vi "Climb_Execute.vi"() -> ()   [LabVIEW 2018]
uses:
  <vilib>/Rock Robotics/WPI/ThirdParty/Phoenix-LabVIEW/Motor Controller/Controls/CTRE_Phoenix_MotorControl_ControlMode.ctl
  <vilib>/Rock Robotics/WPI/Solenoid/WPI_SolenoidValue.ctl
  Global_Variables/Climb_Globals.vi
  <vilib>/Rock Robotics/WPI/Solenoid/WPI_SolenoidGetEnum.vi
  Global_Variables/Sensor_Values.vi
  <vilib>/Rock Robotics/WPI/Solenoid/WPI_SolenoidSetEnum.vi
panel:
  in  "Speed_Down":dbl=-0.3 format="%#_13g"
  in  "Drop_Pos":dbl=2500.0
  in  "Climb_Gain":dbl=0.00012
  in  "Gain":dbl=1e-06
  in  "Backward_Speed":dbl=-1.0
  in  "Forward_Speed":dbl=1.0
  in  "Down_Speed":dbl=-0.3
  in  "Up_Speed":dbl=0.2
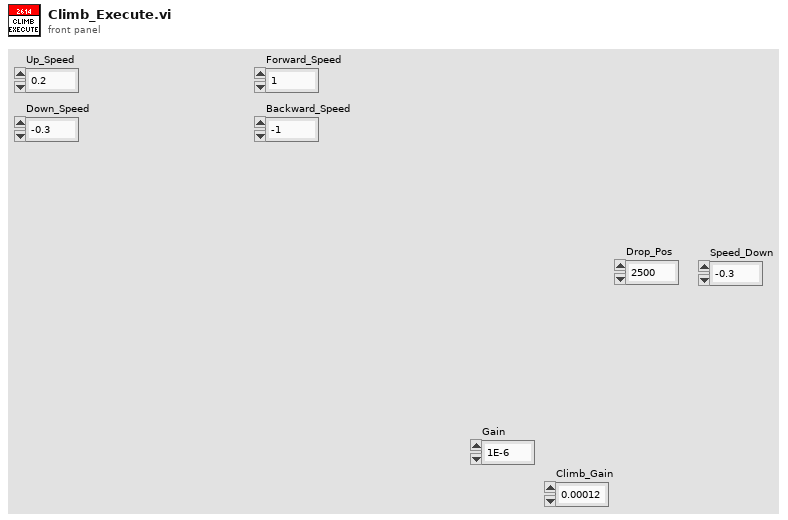
[diagram p1: front panel]
types:
  T1 = typedef "WPI_SolenoidDevRef.ctl" = cluster{"DevStatus":errorcluster, "Pneumatics Control Module":u8, "Forward Solenoid Channel":T2, "Reverse Solenoid Channel":T2}
  T2 = typedef "WPI_SolenoidChannel.ctl" = enum8{"Solenoid 0", "Solenoid 1", "Solenoid 2", "Solenoid 3", "Solenoid 4", "Solenoid 5", "Solenoid 6", "Solenoid 7", "Invalid"}
  T3 = typedef "WPI_SolenoidValue.ctl" = enum16{"Off", "On", "Forward", "Reverse"}
  T4 = typedef "WPI_MotorControlDeviceRef.ctl" = cluster{"DeviceStatus":errorcluster, "Type":T5, "PWM":cluster{"PWM Channel":T6, "DeadBand":T7}, "CAN":cluster{"Device Number":u8, "SetOutput VI Ref":variant, "GetOutput VI Ref":variant, "Enable VI Ref":variant, "Disable VI Ref":variant, "Data":variant}, "Invert":bool, "DIO PWM":cluster{"PWM \"Enable\" Channel":T6, "DIOChannel":T8, "PWM Rate":dbl}}
  T5 = typedef "WPI_MotorControlType.ctl" = enum16{"PWM", "CAN", "DIO PWM"}
  T6 = typedef "FPGA_DIOPWMChannel.ctl" = enum8{"PWM 0", "PWM 1", "PWM 2", "PWM 3", "PWM 4", "PWM 5", "PWM 6", "PWM 7", "PWM 8", "PWM 9", "PWM MXP 0", "PWM MXP 1", "PWM MXP 2", "PWM MXP 3", "PWM MXP 4", "PWM MXP 5", "PWM MXP 6", "PWM MXP 7", "PWM MXP 8", "PWM MXP 9", "Invalid"}
  T7 = typedef "WPI_PWMDeadband.ctl" = cluster{"Name":string, "maxPositivePwm":i32, "minPositivePwm":i32, "centerPwm":i32, "maxNegativePwm":i32, "minNegativePwm":i32, "angularRange":u16}
  T8 = typedef "FPGA_DIOChannel.ctl" = enum8{"DIO 0", "DIO 1", "DIO 2", "DIO 3", "DIO 4", "DIO 5", "DIO 6", "DIO 7", "DIO 8", "DIO 9", "DIO MXP 0", "DIO MXP 1", "DIO MXP 2", "DIO MXP 3", "DIO MXP 4", "DIO MXP 5", "DIO MXP 6", "DIO MXP 7", "DIO MXP 8", "DIO MXP 9", "DIO MXP 10", "DIO MXP 11", "DIO MXP 12", "DIO MXP 13", "DIO MXP 14", "DIO MXP 15", "SPI Port CS1", "SPI Port CS2", "SPI Port CS3", "SPI Port MISO", "SPI Port MOSI", "Invalid"}
  T9 = typedef "WPI_ServoDeviceRef.ctl" = cluster{"DeviceStatus":errorcluster, "PWM Channel":T6, "DeadBand":T7}
  T10 = typedef "Climb_Notifier.ctl" = cluster{"Climb_Control_Type":T11, "Brake":bool, "Manual_Climb_Up":bool, "Manual_Drive_Forward":bool, "Manual_Drive_Backward":bool, "Manual_Climb_Down":bool, "Climb_Advance":bool, "Climb_Reverse":bool, "Parameter_One":dbl, "Parameter_Two":dbl, "Parameter_Three":dbl, "Step":i32, "Climb_Notifier":refnum<notifier>, "Climb_Distance":dbl, "Level_Two":bool, "Brake_State":bool, "Toggle_Servo":bool, "Drop_Back":bool}
  T11 = typedef "Climb_Control_Type.ctl" = enum16{"No_Op", "Brake", "Manual_Climb_Up", "Manual_Climb_Down", "Manual_Drive_Forward", "Manual_Drive_Backward", "Back_Wheels_Forward", "Lift_Retract", "Lift_Extend", "Extend_to_Second_Level", "Drop_Down", "Spin"}
  T12 = typedef "CTRE_Phoenix_MotorControl_ControlMode.ctl" = u16
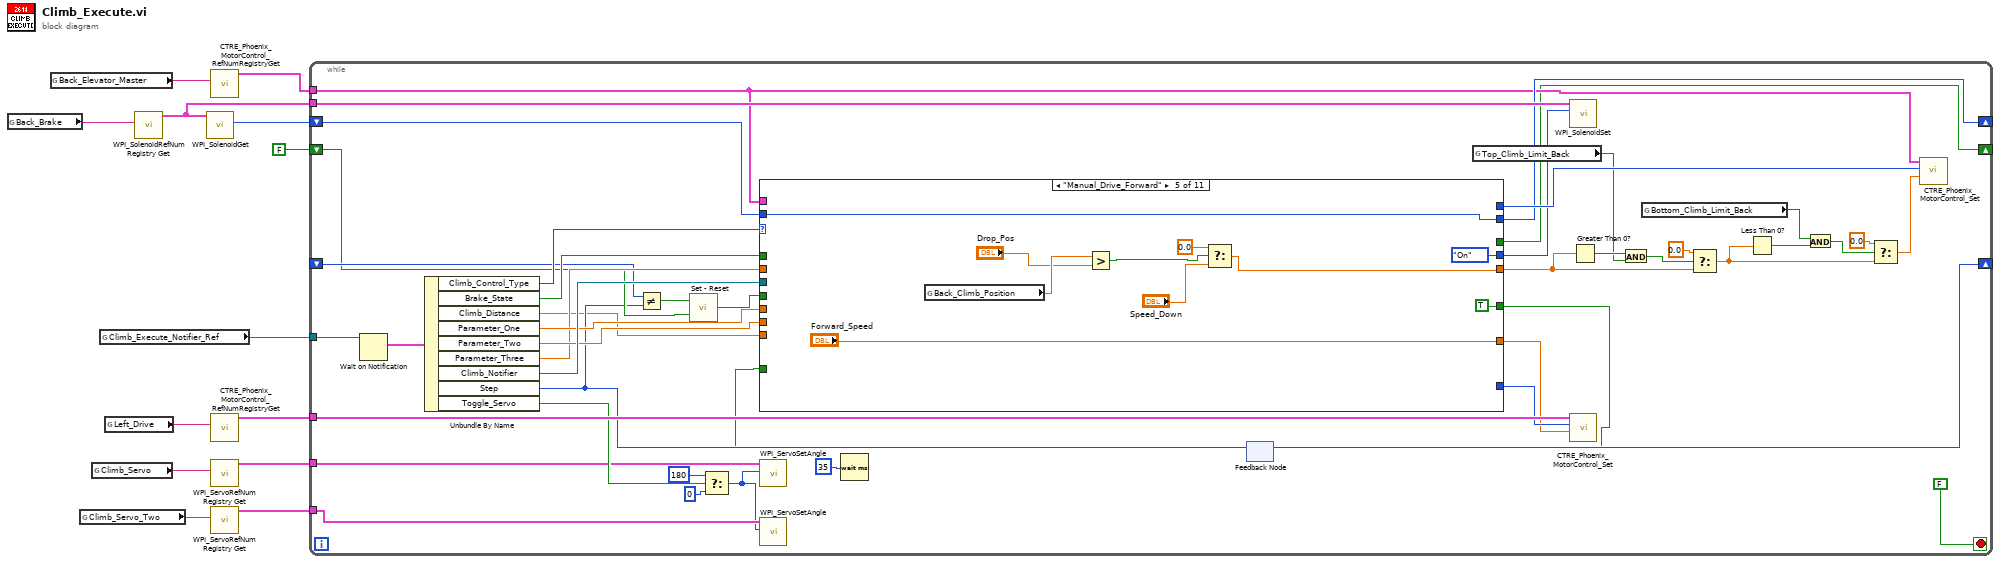
[diagram p0: block diagram]
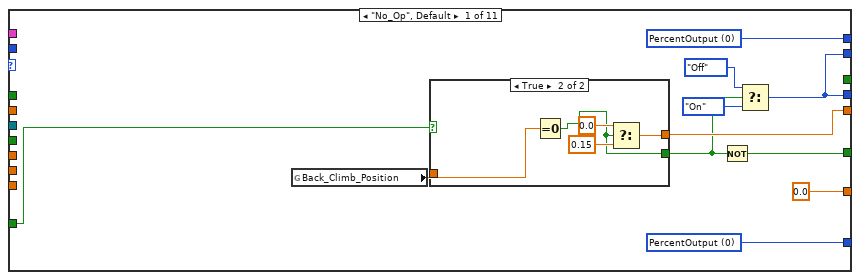
[diagram p2: hidden frame]
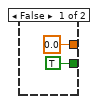
[diagram p3: hidden frame]
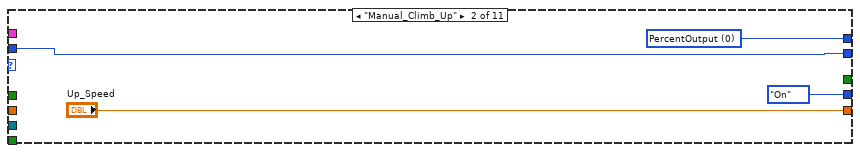
[diagram p4: hidden frame]
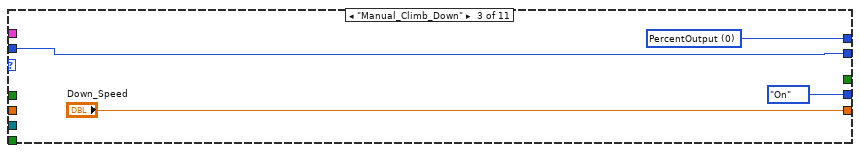
[diagram p5: hidden frame]
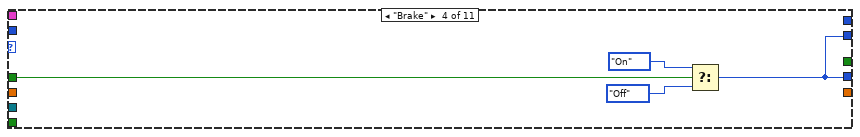
[diagram p6: hidden frame]
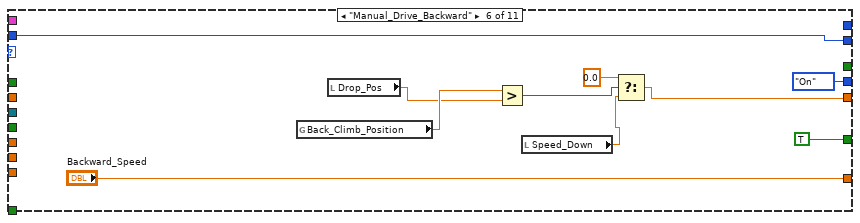
[diagram p7: hidden frame]
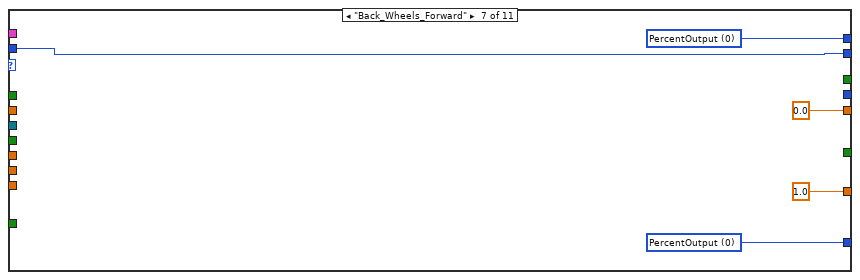
[diagram p8: hidden frame]
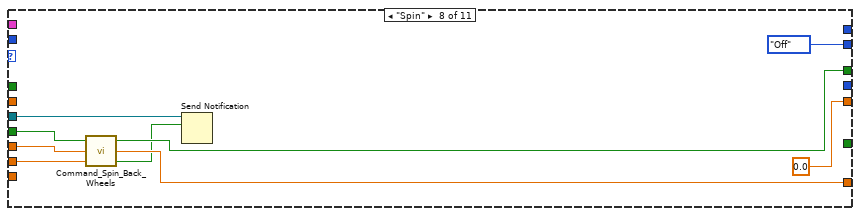
[diagram p9: hidden frame]
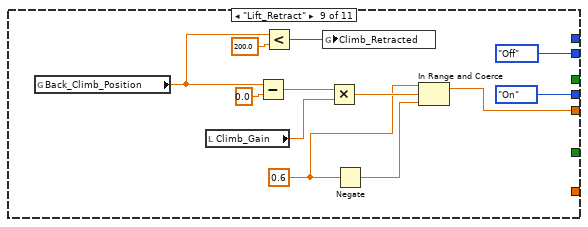
[diagram p10: hidden frame]
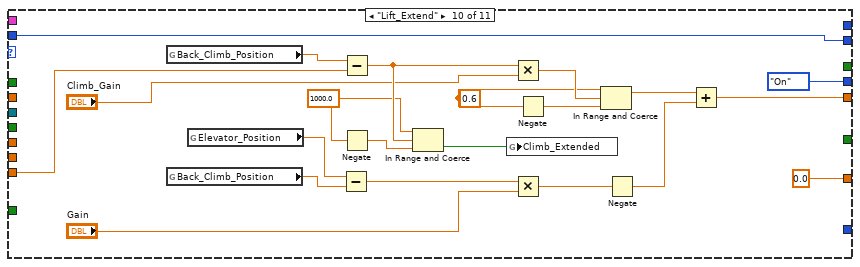
[diagram p11: hidden frame]
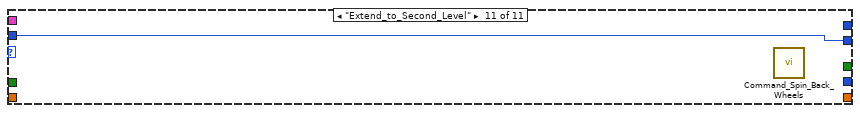
[diagram p12: hidden frame]
diagram:
  n1 = global read "Climb_Globals.vi" "Back_Brake"() -> (w8:string)
  n2 = global read "Climb_Globals.vi" "Back_Elevator_Master"() -> (w11:string)
  n3 = global read "Climb_Globals.vi" "Climb_Servo_Two"() -> (w2:string)
  n4 = global read "Climb_Globals.vi" "Climb_Servo"() -> (w3:string)
  n5 = global read "Climb_Globals.vi" "Climb_Execute_Notifier_Ref"() -> (w12:refnum<notifier>)
  n6 = global read "Climb_Globals.vi" "Left_Drive"() -> (w10:string)
  n7 = call <vilib>:"WPI_SolenoidRefNum Registry Get.vi"("refnum name"=w8) -> ("SolenoidDevRef"=w5:T1)  [unwired: 9 in, 1 out]
  n8 = call-poly <vilib>:"WPI_SolenoidGet.vi"("SolenoidDevRef"=w5) -> ("Value"=w6:T3)  [unwired: 8 in, 2 out]
  n9 = call <vilib>:"CTRE_Phoenix_MotorControl_RefNumRegistryGet.vi"("refnum name"=w11) -> ("PhoenixMotorControlDevRef"=w13:T4)  [unwired: 9 in, 1 out]
  n10 = call <vilib>:"CTRE_Phoenix_MotorControl_RefNumRegistryGet.vi"("refnum name"=w10) -> ("PhoenixMotorControlDevRef"=w9:T4)  [unwired: 9 in, 1 out]
  n11 = call <vilib>:"WPI_ServoRefNum Registry Get.vi"("refnum name"=w3) -> ("ServoDeviceRef"=w4:T9)  [unwired: 9 in, 1 out]
  n12 = call <vilib>:"WPI_ServoRefNum Registry Get.vi"("refnum name"=w2) -> ("ServoDeviceRef"=w1:T9)  [unwired: 9 in, 1 out]
  n13 = while {
    tunnel: w12 -> [w56]
    tunnel: w13 -> [w35]
    tunnel: w9 -> [w53]
    tunnel: w5 -> [w51]
    shift-right: [w49] -> _
    shift-left: w6 -> [w48]
    shift-right: [w25] -> _
    shift-left: _ -> [w28]
    shift-right: [w23] -> _
    shift-left: FALSE -> [w26]
    tunnel: w4 -> [w19]
    tunnel: w1 -> [w17]
    stop <- FALSE stop-if-true
    n14 = Wait on Notification(notifier=w56) -> (notification=w55:T10)  [unwired: 3 in, 3 out]
    n15 = Unbundle By Name(w55) -> ("Climb_Control_Type"=w33:T11, "Brake_State"=w47:bool, "Climb_Distance"=w22:dbl, "Parameter_One"=w31:dbl, "Parameter_Two"=w30:dbl, "Parameter_Three"=w29:dbl, "Climb_Notifier"=w32:refnum<notifier>, "Step"=w25:i32, "Toggle_Servo"=w21:bool)
    n16 = Not Equal?(x=w28, y=w25) -> (x != y?=w27:bool)
    n17 = call "Set - Reset.vi"("Reset"=w26, "Set"=w27) -> ("Output"=w24:bool)
    n18 = Select(t=180, s=w21, f=0 ("Angle")) -> (s? t:f=w16:i32)
    n19 = call <vilib>:"WPI_ServoSetAngle.vi"("Angle"=w16, "ServoDeviceRef"=w19) -> ()  [unwired: 8 in, 2 out]
    n20 = call <vilib>:"WPI_ServoSetAngle.vi"("Angle"=w16, "ServoDeviceRef"=w17) -> ()  [unwired: 8 in, 2 out]
    n21 = Wait (ms)(milliseconds to wait=u32 35) -> ()  [unwired: 1 out]
    n22 = feedback #1() -> (w14:bool)  [unwired: 1 in]
    n23 = case shown="\"Manual_Drive_Forward\"" w33 {
      tunnel: [w69 w78 w82 _ _ _ w112 _ _ _ _] -> w54
      tunnel: [w68 _ _ _ _ _ w111 _ _ _ _] -> w52
      tunnel: [0.0 ("Output") _ _ _ "Forward_Speed" "Backward_Speed" 1.0 ("Speed") w118 _ 0.0 ("Speed") _] -> w38
      tunnel: [w63 WPI_SolenoidValue."On" ("Value") WPI_SolenoidValue."On" ("Value") w86 WPI_SolenoidValue."On" ("Value") WPI_SolenoidValue."On" ("Value") _ _ WPI_SolenoidValue."On" ("Value") WPI_SolenoidValue."On" ("Value") _] -> w50
      tunnel: w47 -> [_ _ _ w85 _ _ _ _ _ _ _]
      tunnel: [w63 w80 w84 w86 w97 w107 w113 WPI_SolenoidValue."Off" ("Value") WPI_SolenoidValue."Off" ("Value") w136 w156] -> w49
      tunnel: w48 -> [_ w80 w84 _ w97 w107 w113 _ _ w136 w156]
      tunnel: w35 -> [_ _ _ _ _ _ _ _ _ _ _]
      tunnel: [w65 "Up_Speed" "Down_Speed" _ w94 w105 0.0 ("upper limit") 0.0 ("upper limit") w125 w142 _] -> w34
      tunnel: w32 -> [_ _ _ _ _ _ _ w114 _ _ _]
      tunnel: w31 -> [_ _ _ _ _ _ _ w121 _ _ _]
      tunnel: w30 -> [_ _ _ _ _ _ _ w120 _ _ _]
      tunnel: w29 -> [_ _ _ _ _ _ _ _ _ _ _]
      tunnel: w24 -> [_ _ _ _ _ _ _ w119 _ _ _]
      tunnel: [_ _ _ _ _ _ _ w116 _ _ _] -> w23
      tunnel: w22 -> [_ _ _ _ _ _ _ _ _ w135 _]
      tunnel: [w59 _ _ _ TRUE TRUE _ _ _ _ _] -> w15
      tunnel: w14 -> [w64 _ _ _ _ _ _ _ _ _ _]
      frame "No_Op", Default {
        w68 = T12 0 items=["PercentOutput"=0, "Position"=1, "Velocity"=2, "Current"=3, "Follower"=5, "MotionProfile"=6, "MotionMagic"=7, "MotionProfileArc"=10, "Disabled"=15] ("Control Mode")
        w69 = T12 0 items=["PercentOutput"=0, "Position"=1, "Velocity"=2, "Current"=3, "Follower"=5, "MotionProfile"=6, "MotionMagic"=7, "MotionProfileArc"=10, "Disabled"=15] ("Control Mode")
        n24 = global read "Sensor_Values.vi" "Back_Climb_Position"() -> (w66:dbl)
        n25 = case shown="True" w64 {
          tunnel: w66 -> [_ w73]
          tunnel: [0.0 ("f") w74] -> w65
          tunnel: [TRUE w72] -> w62
          frame False {
          }
          frame True {
            n26 = Equal To 0?(x=w73) -> (x = 0?=w72:bool)
            n27 = Select(t=0.0, s=w72, f=0.15) -> (s? t:f=w74:dbl)
          }
        }
        n28 = Not(x=w62) -> (.not. x?=w59:bool)
        n29 = Select(t=WPI_SolenoidValue."Off" ("Value"), s=w62, f=WPI_SolenoidValue."On") -> (s? t:f=w63:T3)
      }
      frame "Manual_Climb_Up" {
        w78 = T12 0 items=["PercentOutput"=0, "Position"=1, "Velocity"=2, "Current"=3, "Follower"=5, "MotionProfile"=6, "MotionMagic"=7, "MotionProfileArc"=10, "Disabled"=15] ("Control Mode")
      }
      frame "Manual_Climb_Down" {
        w82 = T12 0 items=["PercentOutput"=0, "Position"=1, "Velocity"=2, "Current"=3, "Follower"=5, "MotionProfile"=6, "MotionMagic"=7, "MotionProfileArc"=10, "Disabled"=15] ("Control Mode")
      }
      frame "Brake" {
        n30 = Select(t=WPI_SolenoidValue."On" ("Value"), s=w85, f=WPI_SolenoidValue."Off" ("Value")) -> (s? t:f=w86:T3)
      }
      frame "Manual_Drive_Forward" {
        n31 = global read "Sensor_Values.vi" "Back_Climb_Position"() -> (w91:dbl)
        n32 = Greater?(x=w91, y="Drop_Pos") -> (0:w89:bool)
        n33 = Select(t=0.0, s=w89, f="Speed_Down") -> (s? t:f=w94:dbl)
      }
      frame "Manual_Drive_Backward" {
        n34 = global read "Sensor_Values.vi" "Back_Climb_Position"() -> (w101:dbl)
        n35 = local read "Drop_Pos"() -> (w99:dbl)
        n36 = Greater?(x=w101, y=w99) -> (0:w100:bool)
        n37 = local read "Speed_Down"() -> (w102:dbl)
        n38 = Select(t=0.0, s=w100, f=w102) -> (s? t:f=w105:dbl)
      }
      frame "Back_Wheels_Forward" {
        w111 = T12 0 items=["PercentOutput"=0, "Position"=1, "Velocity"=2, "Current"=3, "Follower"=5, "MotionProfile"=6, "MotionMagic"=7, "MotionProfileArc"=10, "Disabled"=15] ("Control Mode")
        w112 = T12 0 items=["PercentOutput"=0, "Position"=1, "Velocity"=2, "Current"=3, "Follower"=5, "MotionProfile"=6, "MotionMagic"=7, "MotionProfileArc"=10, "Disabled"=15] ("Control Mode")
      }
      frame "Spin" {
        n39 = call "Command_Spin_Back_Wheels.vi"("Timeout"=w120, "Speed"=w121, "Startup"=w119) -> ("Completed"=w115:bool, "Speed_Out"=w118:dbl, "Reinit"=w116:bool)
        n40 = Send Notification(notification=w115, notifier=w114) -> ()  [unwired: 1 in, 2 out]
      }
      frame "Lift_Retract" {
        w129 = 0.6 ("upper limit")
        n41 = global read "Sensor_Values.vi" "Back_Climb_Position"() -> (w127:dbl)
        n42 = local read "Climb_Gain"() -> (w133:dbl)
        n43 = Subtract(x=w127, y=0.0) -> (x-y=w134:dbl)
        n44 = Less?(x=w127, y=200.0) -> (x < y?=w126:bool)
        n45 = global write "Climb_Globals.vi" "Climb_Retracted"(w126) -> ()
        n46 = Multiply(x=w134, y=w133) -> (x*y=w132:dbl)
        n47 = Negate(x=w129) -> (-x=w131:dbl)
        n48 = In Range and Coerce(upper limit=w129, x=w132, lower limit=w131) -> (coerced(x)=w125:dbl)  [unwired: 1 out]
      }
      frame "Lift_Extend" {
        w140 = 1000.0 ("upper limit")
        w139 = 0.6 ("upper limit")
        n49 = global read "Sensor_Values.vi" "Back_Climb_Position"() -> (w153:dbl)
        n50 = global read "Sensor_Values.vi" "Back_Climb_Position"() -> (w147:dbl)
        n51 = global read "Sensor_Values.vi" "Elevator_Position"() -> (w146:dbl)
        n52 = Subtract(x=w146, y=w147) -> (x-y=w145:dbl)
        n53 = Subtract(x=w153, y=w135) -> (x-y=w155:dbl)
        n54 = Negate(x=w140) -> (-x=w154:dbl)
        n55 = In Range and Coerce(upper limit=w140, x=w155, lower limit=w154) -> (In Range?=w141:bool)  [unwired: 1 out]
        n56 = global write "Climb_Globals.vi" "Climb_Extended"(w141) -> ()
        n57 = Multiply(x=w155, y="Climb_Gain") -> (x*y=w150:dbl)
        n58 = Multiply(x=w145, y="Gain") -> (x*y=w144:dbl)
        n59 = Negate(x=w139) -> (-x=w149:dbl)
        n60 = In Range and Coerce(upper limit=w139, x=w150, lower limit=w149) -> (coerced(x)=w152:dbl)  [unwired: 1 out]
        n61 = Negate(x=w144) -> (-x=w148:dbl)
        n62 = Add(x=w152, y=w148) -> (x+y=w142:dbl)
      }
      frame "Extend_to_Second_Level" {
        n63 = call "Command_Spin_Back_Wheels.vi"() -> ()  [unwired: 3 in, 3 out]
      }
    }
    n64 = feedback-in #1(w15) -> ()
    n65 = global read "Sensor_Values.vi" "Top_Climb_Limit_Back"() -> (w45:bool)
    n66 = call-poly <vilib>:"WPI_SolenoidSet.vi"("Value"=w50, "SolenoidDevRef"=w51) -> ()  [unwired: 8 in, 2 out]
    n67 = call <vilib>:"CTRE_Phoenix_MotorControl_Set.vi"("Output"=w38, "Control Mode"=w52, "PhoenixMotorControlDevRef"=w53) -> ()  [unwired: 7 in, 2 out]
    n68 = Greater Than 0?(x=w34) -> (x > 0?=w46:bool)
    n69 = And(x=w46, y=w45) -> (x .and. y?=w44:bool)
    n70 = global read "Sensor_Values.vi" "Bottom_Climb_Limit_Back"() -> (w40:bool)
    n71 = Select(t=0.0, s=w44, f=w34) -> (s? t:f=w36:dbl)
    n72 = Less Than 0?(x=w36) -> (x < 0?=w39:bool)
    n73 = And(x=w40, y=w39) -> (x .and. y?=w41:bool)
    n74 = Select(t=0.0, s=w41, f=w36) -> (s? t:f=w37:dbl)
    n75 = call <vilib>:"CTRE_Phoenix_MotorControl_Set.vi"("Output"=w37, "Control Mode"=w54, "PhoenixMotorControlDevRef"=w35) -> ()  [unwired: 7 in, 2 out]
  }
